vi "Check User Exist.vi"(7 "PwdMgr in":refnum<class "PwdMgr.lvclass">, 8 "Error in":errorcluster caption="Error in (no error)", 11 "Username":string) -> (0 "Error out":errorcluster, 2 "exist？":bool, 3 "Username":string)   [LabVIEW 2020, in "Login-UI.lvlib" / "PwdMgr.lvclass"]
uses:
  PwdMgr/PwdMgr.lvclass
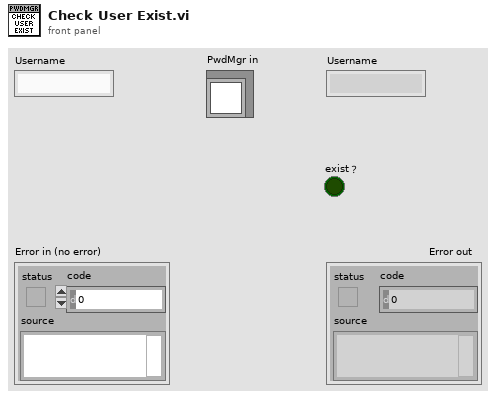
[diagram p1: front panel]
types:
  T1 = typedef "Login-UI.lvlib/User-Info.ctl" = cluster{"UserName":string, "Password":string, "Role":T2}
  T2 = typedef "Login-UI.lvlib/User-Role.ctl" = enum16{"INVALID", "Operator", "Engineer", "Admin", "Anonymous"}
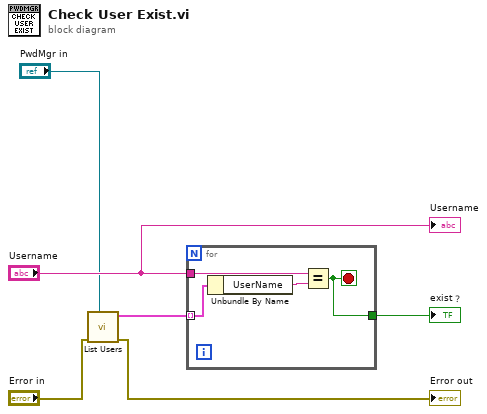
[diagram p0: block diagram]
diagram:
  n1 = call-dynamic "List Users.vi"("PwdMgr in"="PwdMgr in", "error in (no error)"="Error in") -> ("error out"=→"Error out":errorcluster, "Array"=w6:T1[])  [unwired: 8 in]
  n2 = for {
    tunnel: w6 -> [w8] mode=indexing
    tunnel: "Username" -> [w10]
    tunnel: [w7] -> w2
    stop <- w7 stop-if-true
    n3 = Unbundle By Name(w8) -> ("UserName"=w9:string)
    n4 = Equal?(x=w10, y=w9) -> (x = y?=w7:bool)
  }
  "exist？" <- w2
  "Username" <- "Username"
